vi "Panel Resized.vi"(6 "Sizing Refnums":T2, 8 "error in (no error)":errorcluster, 9 "Origin":cluster{"H":i16, "V":i16}, 10 "NewBnds":T1, 11 "Size Constraints":cluster{"min tab width":i32, "w/h":dbl}) -> (0 "error out":errorcluster)   [LabVIEW 2015]
uses:
  <vilib>/Utility/miscctls.llb/LVRectTypeDef.ctl
  <vilib>/Utility/miscctls.llb/LVRowAndColumnTypeDef.ctl
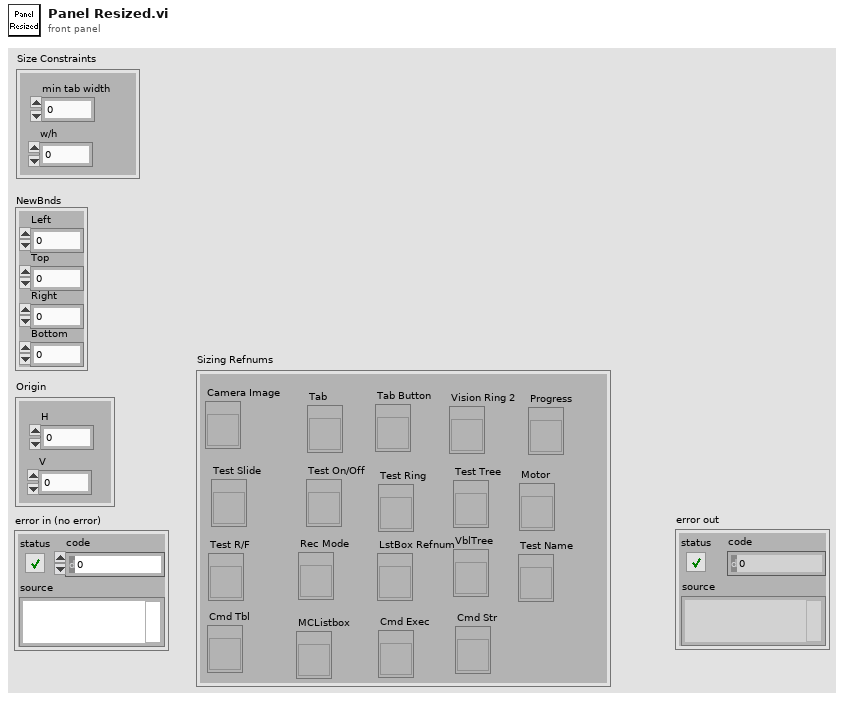
[diagram p1: front panel]
types:
  T1 = typedef "LVRectTypeDef.ctl" = cluster{"Left":i16, "Top":i16, "Right":i16, "Bottom":i16}
  T2 = cluster{"Camera Image":refnum<vi>, "Tab":refnum<vi>, "Tab Button":refnum<vi>, "Vision Ring 2":refnum<vi>, "Rec Mode":refnum<vi>, "Test Slide":refnum<vi>, "Test On/Off":refnum<vi>, "Test Ring":refnum<vi>, "Test R/F":refnum<vi>, "Test Name":refnum<vi>, "Motor":refnum<vi>, "Progress":refnum<vi>, "LstBox Refnum":refnum<vi>, "Test Tree":refnum<vi>, "VblTree":refnum<vi>, "Cmd Tbl":refnum<vi>, "MCListbox":refnum<vi>, "Cmd Exec":refnum<vi>, "Cmd Str":refnum<vi>}
  T3 = typedef "LVRowAndColumnTypeDef.ctl" = cluster{"Row":i32, "Column":i32}
  T4 = typedef "LVPositionTypeDef.ctl" = cluster{"Left":i32, "Top":i32}
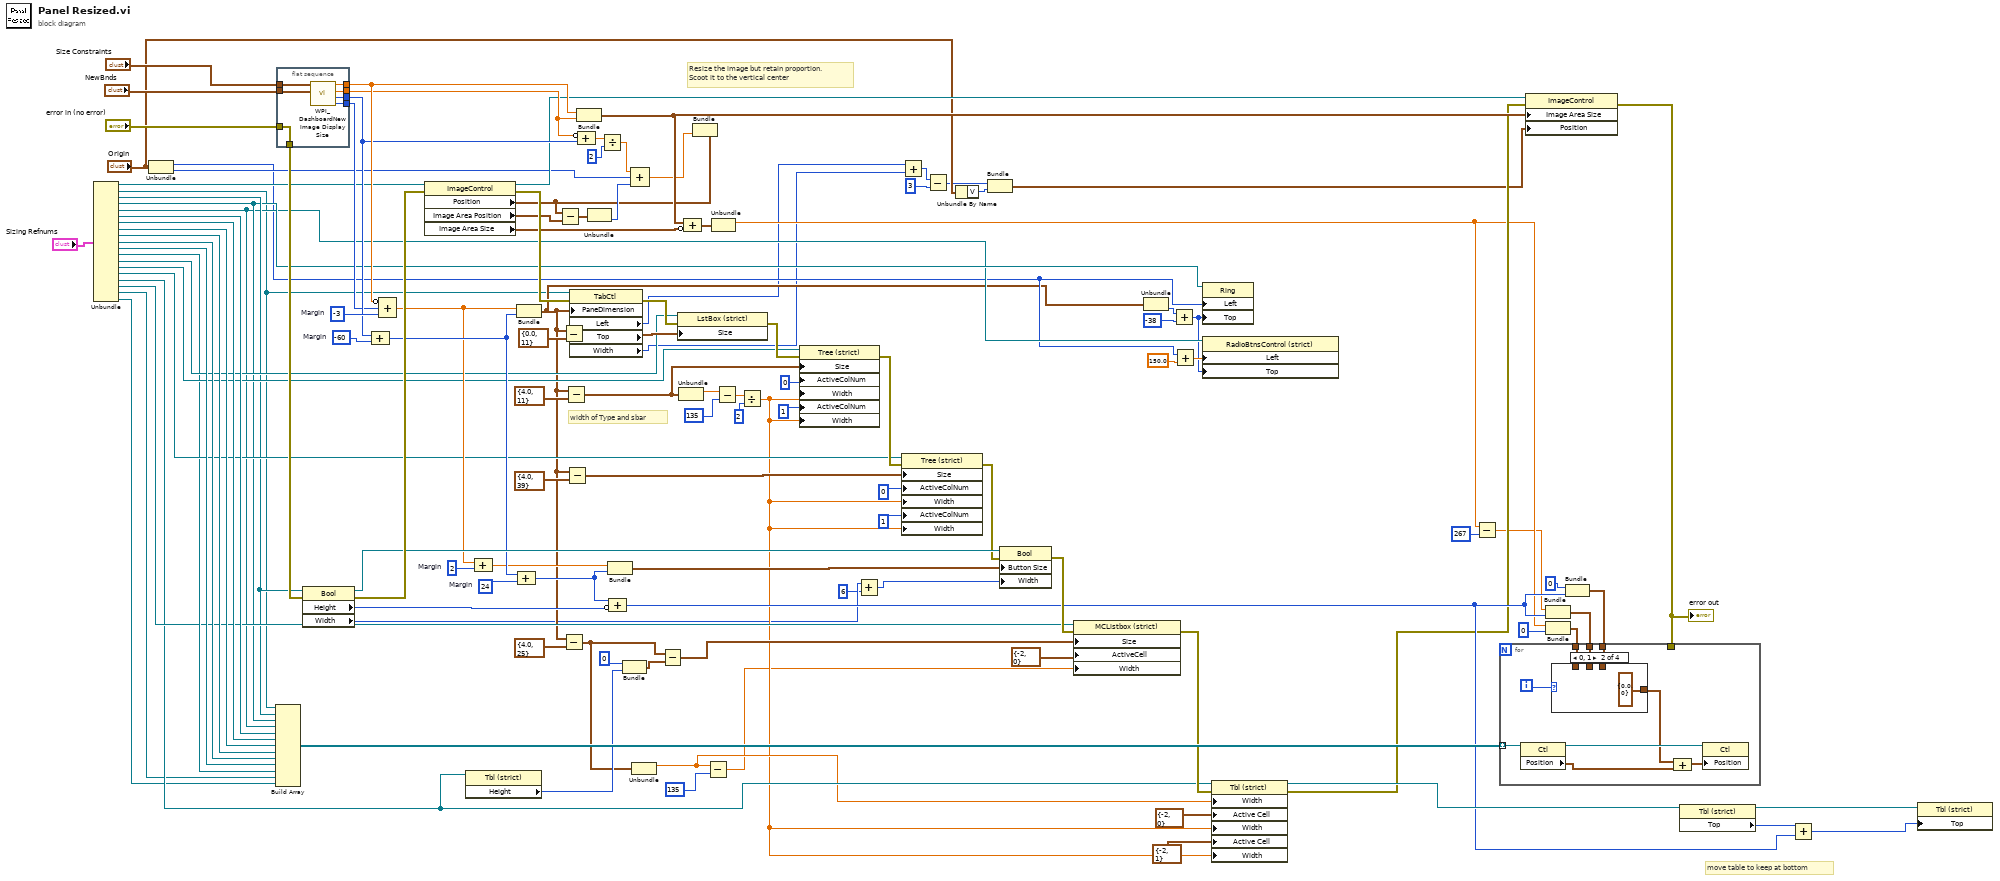
[diagram p0: block diagram]
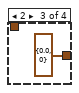
[diagram p3: hidden frame]
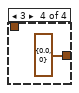
[diagram p4: hidden frame]
diagram:
  w105 = 24  # Margin
  w103 = 2  # Margin
  w99 = -60  # Margin
  w109 = -3  # Margin
  # "move table to keep at bottom"
  # "width of Type and sbar"
  # "Resize the image but retain proportion.\nScoot it to the vertical center"
  n1 = Unbundle("Sizing Refnums") -> ("Camera Image"=w77:refnum<vi>, "Tab"=w6:refnum<vi>, "Tab Button"=w25:refnum<vi>, "Vision Ring 2"=w19:refnum<vi>, "Rec Mode"=w18:refnum<vi>, "Test Slide"=w118:refnum<vi>, "Test On/Off"=w119:refnum<vi>, "Test Ring"=w120:refnum<vi>, "Test R/F"=w121:refnum<vi>, "Test Name"=w58:refnum<vi>, "Motor"=w57:refnum<vi>, "Progress"=w51:refnum<vi>, "LstBox Refnum"=w52:refnum<vi>, "Test Tree"=w53:refnum<vi>, "VblTree"=w54:refnum<vi>, "Cmd Tbl"=w45:refnum<vi>, "MCListbox"=w46:refnum<vi>, "Cmd Exec"=w27:refnum<vi>, "Cmd Str"=w26:refnum<vi>)
  n2 = Unbundle("Origin") -> ("H"=w14:i16, "V"=w82:i16)
  n3 = Build Array(w6, w25, w19, w18, w118, w119, w120, w121, w58, w57, w51, w27, w26) -> (w117:refnum<vi>[])
  n4 = flat-sequence {
    tunnel: "NewBnds" -> [w128]
    tunnel: "Size Constraints" -> [w127]
    tunnel: [w126] -> w98
    tunnel: [w125] -> w106
    tunnel: [w124] -> w107
    tunnel: [w123] -> w108
    tunnel: [w122] -> w116
    tunnel: "error in (no error)" -> [w122]
    frame #0 {
      n5 = call <vilib>:"WPI_DashboardNew Image Display Size.vi"("NewBnds"=w128, "Size Constraints"=w127) -> ("Window Width"=w126:i16, "Window Height"=w124:i16, "Height"=w125:dbl, "Width"=w123:dbl)  [unwired: 6 in]
    }
  }
  n6 = property class="Bool"(reference=w25, error in=w116) -> (reference out=w112:refnum<vi>, error out=w115:errorcluster, "Height"=w111:u32, "Width"=w2:u32)
  n7 = Compound Arithmetic op=unknown(w107, w99) -> (w104:i32)
  n8 = Compound Arithmetic op=ADD(invert w108, w98, w109) -> (w102:dbl)
  n9 = property class="ImageControl"(reference=w77, error in=w115) -> (reference out=w92:refnum<vi>, error out=w114:errorcluster, "Position"=w91:T4, "Image Area Position"=w86:cluster{"Left":i32, "Top":i32}, "Image Area Size"=w96:cluster{"Width":u32, "Height":u32})
  n10 = property class="Tbl (strict)"(reference=w45) -> ("Height"=w44:u32)  [unwired: 1 in, 2 out]
  n11 = Compound Arithmetic op=ADD(w102, w103) -> (w101:dbl)
  n12 = Bundle(w102, w104) -> (w13:cluster{dbl, i32})  [unwired: 1 in]
  n13 = Compound Arithmetic op=ADD(w104, w105) -> (w110:i32)
  n14 = Subtract(x=w91, y=w86) -> (x-y=w93:T4)
  n15 = Subtract(x=w13, y=cluster{dbl, i32} {0.0, 11}) -> (x-y=w75:cluster{dbl, i32})
  n16 = Subtract(x=w13, y=cluster{dbl, i32} {4.0, 25}) -> (x-y=w41:cluster{dbl, i32})
  n17 = Subtract(x=w13, y=cluster{dbl, i32} {4.0, 11}) -> (x-y=w65:cluster{dbl, i32})
  n18 = Subtract(x=w13, y=cluster{dbl, i32} {4.0, 39}) -> (x-y=w71:cluster{dbl, i32})
  n19 = property class="TabCtl" props=["PaneDimension", "Left", "Top", "Width"](reference=w6, error in=w114, "PaneDimension"=w13) -> (error out=w76:errorcluster, "Left"=w5:i32, "Width"=w4:u32)  [unwired: 2 out]
  n20 = Bundle("Width"=w108, "Height"=w106) -> (w95:cluster{"Width":dbl, "Height":dbl})  [unwired: 1 in]
  n21 = Compound Arithmetic op=ADD(invert w106, w107) -> (w87:dbl)
  n22 = Unbundle(w93) -> ("Top"=w94:i32)  [unwired: 1 out]
  n23 = Divide(x=w87, y=2) -> (x/y=w89:dbl)
  n24 = Bundle(w101, w110) -> (w100:cluster{dbl, i32})  [unwired: 1 in]
  n25 = Compound Arithmetic op=ADD(w110, invert w111) -> (w36:u32)
  n26 = Bundle(0, "Height"=w44) -> (w42:cluster{i32, "Height":u32})  [unwired: 1 in]
  n27 = Compound Arithmetic op=ADD(w89, w82, w94) -> (w90:dbl)
  n28 = Unbundle(w41) -> (w31:dbl)  [unwired: 1 out]
  n29 = Subtract(x=w41, y=w42) -> (x-y=w40:cluster{dbl, u32})
  n30 = property class="LstBox (strict)"(reference=w52, error in=w76, "Size"=w75) -> (error out=w70:errorcluster)  [unwired: 1 out]
  n31 = Unbundle(w65) -> (w64:dbl)  [unwired: 1 out]
  n32 = Compound Arithmetic op=ADD(w95, invert w96) -> (w97:cluster{"Width":dbl, "Height":dbl})
  n33 = Bundle(cluster=w91, "Top"=w90) -> ()  [unwired: 1 in, 1 out]
  n34 = Subtract(x=w31, y=135) -> (x-y=w28:dbl)
  n35 = Unbundle(w97) -> ("Width"=w23:dbl)  [unwired: 1 out]
  n36 = Subtract(x=w64, y=135 ("Active Cell:Active Column Number")) -> (x-y=w60:dbl)
  n37 = Divide(x=w60, y=2 ("Active Cell:Active Column Number")) -> (x/y=w29:dbl)
  n38 = property class="Tree (strict)"(reference=w53, error in=w70, "Size"=w65, "ActiveColNum"=0 ("Active Cell:Active Column Number"), "Width"=w29, "ActiveColNum"=1 ("Active Cell:Active Column Number"), "Width"=w29) -> (error out=w69:errorcluster)  [unwired: 1 out]
  n39 = Add(x=w2, y=u32 6) -> (x+y=w3:u32)
  n40 = Add(x=w5, y=w4) -> (x+y=w21:u32)
  n41 = property class="Tree (strict)"(reference=w54, error in=w69, "Size"=w71, "ActiveColNum"=0 ("Active Cell:Active Column Number"), "Width"=w29, "ActiveColNum"=1 ("Active Cell:Active Column Number"), "Width"=w29) -> (error out=w68:errorcluster)  [unwired: 1 out]
  n42 = Subtract(x=w21, y=u32 3) -> (x-y=w8:u32)
  n43 = Unbundle By Name("Origin") -> ("V"=w7:i16)
  n44 = Bundle(w8, "V"=w7) -> (w9:cluster{u32, "V":i16})  [unwired: 1 in]
  n45 = property class="Bool"(reference=w112, error in=w68, "Button Size"=w100, "Width"=w3) -> (error out=w50:errorcluster)  [unwired: 1 out]
  n46 = property class="MCListbox (strict)"(reference=w46, error in=w50, "Size"=w40, "ActiveCell"=T3 {"Row"=-2, "Column"=0} ("Active Cell:Active Cell"), "Width"=w28) -> (error out=w47:errorcluster)  [unwired: 1 out]
  n47 = Unbundle(w13) -> (w12:i32)  [unwired: 1 out]
  n48 = Add(x=w12, y=-38) -> (x+y=w10:i32)
  n49 = Add(x=w14, y=150.0) -> (x+y=w16:dbl)
  n50 = property class="Ring"(reference=w19, "Left"=w14, "Top"=w10) -> ()  [unwired: 1 in, 2 out]
  n51 = property class="RadioBtnsControl (strict)"(reference=w18, "Left"=w16, "Top"=w10) -> ()  [unwired: 1 in, 2 out]
  n52 = property class="Tbl (strict)"(reference=w45, error in=w47, "Width"=w31, "Active Cell"=T3 {"Row"=-2, "Column"=0} ("Active Cell:Active Cell"), "Width"=w29, "Active Cell"=T3 {"Row"=-2, "Column"=1} ("Active Cell:Active Cell"), "Width"=w29) -> (reference out=w39:refnum<vi>, error out=w34:errorcluster)
  n53 = Subtract(x=w23, y=267) -> (x-y=w17:dbl)
  n54 = property class="ImageControl"(reference=w92, error in=w34, "Image Area Size"=w95, "Position"=w9) -> (error out=w81:errorcluster)  [unwired: 1 out]
  "error out" <- w81
  n55 = Bundle(w17, w36) -> (w85:cluster{dbl, u32})  [unwired: 1 in]
  n56 = Bundle("Width"=w23, 0) -> (w84:cluster{"Width":dbl, i32})  [unwired: 1 in]
  n57 = Bundle(0, w36) -> (w55:cluster{i32, u32})  [unwired: 1 in]
  n58 = for {
    tunnel: w117 -> [w137] mode=indexing
    tunnel: w85 -> [w131]
    tunnel: w84 -> [w132]
    tunnel: w81 -> [_]
    tunnel: w55 -> [w130]
    i -> [w133]
    n59 = property class="Ctl"(reference=w137) -> (reference out=w136:refnum<vi>, "Position"=w135:T4)  [unwired: 1 in, 1 out]
    n60 = case shown="0, 1" w133 {
      tunnel: w132 -> [_ _ _ _]
      tunnel: w131 -> [_ _ _ _]
      tunnel: w130 -> [w138 _ _ _]
      tunnel: [w138 cluster{"Width":dbl, u32} {"Width"=0.0, 0} cluster{"Width":dbl, u32} {"Width"=0.0, 0} cluster{"Width":dbl, u32} {"Width"=0.0, 0}] -> w129
      frame Default {
      }
      frame 0, 1 {
      }
      frame 2 {
      }
      frame 3 {
      }
    }
    n61 = Compound Arithmetic op=ADD(w129, w135) -> (w134:cluster{dbl, u32})
    n62 = property class="Ctl"(reference=w136, "Position"=w134) -> ()  [unwired: 1 in, 2 out]
  }
  n63 = property class="Tbl (strict)"(reference=w39) -> (reference out=w38:refnum<vi>, "Top"=w37:i32)  [unwired: 1 in, 1 out]
  n64 = Add(x=w37, y=w36) -> (x+y=w35:u32)
  n65 = property class="Tbl (strict)"(reference=w38, "Top"=w35) -> ()  [unwired: 1 in, 2 out]
